vi "(SubVI)System Command_Set Chip Information.vi"(8 "error in (no error)":errorcluster caption="에러 입력(에러 없음)", 10 "I2C ID":u8 format="%02x", 11 "Chip Type":T1) -> (0 "error out":errorcluster caption="에러 출력", 3 "Read Data":u8[](array[numeric]))   [LabVIEW 2020]
uses:
  Libraries/Haptic IC Class/Haptic IC/Controls/(Ctrl)IC Type.ctl
  Serial/Controls/(Ctrl)Serial_Write Read Option.ctl
  Serial/Instance VIs/(SubVI)Serial_Write-Read.vi
  Libraries/Haptic IC Class/Haptic IC/Haptic IC.lvclass
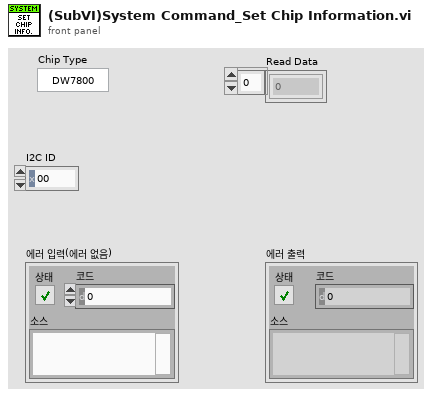
[diagram p1: front panel]
types:
  T1 = typedef "Haptic IC.lvclass/(Ctrl)IC Type.ctl" = enum8{"DW7800", "DW7802", "DW7912", "DW7914"}
  T2 = typedef "(Ctrl)Serial_Write Read Option.ctl" = cluster{"Echo Request":bool, "Header Verification":bool, "Checksum Verification":bool, "User Code Verifiaction":bool}
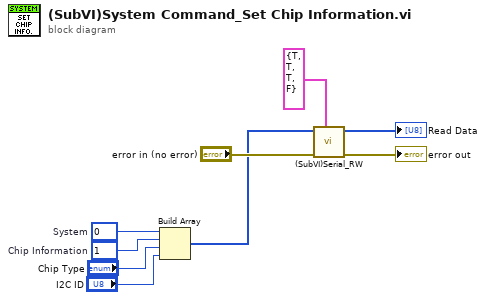
[diagram p0: block diagram]
diagram:
  w7 = u8 1  # Chip Information
  w8 = u8 0  # System
  n1 = Build Array(w8, w7, "Chip Type", "I2C ID") -> (w2:u8[])
  n2 = call-poly "(SubVI)Serial_RW.vi"("Option"=T2 {"Echo Request"=TRUE, "Header Verification"=TRUE, "Checksum Verification"=TRUE, "User Code Verifiaction"=FALSE}, "error in (no error)"="error in (no error)", "Data to Write"=w2) -> ("error out"=→"error out":errorcluster, "Read Data"=→"Read Data":u8[])  [unwired: 6 in, 1 out]
